vi "getItems.vi"(8 "error in (no error)":errorcluster, 11 "IFolder in":refnum<class "IFolder.lvclass">) -> (0 "error out":errorcluster, 2 "Components out":refnum<class "IComponent.lvclass">[](array[class]), 3 "IFolder out":refnum<class "IFolder.lvclass">)   [LabVIEW 2022 SP3, in "openDAQ.lvlib" / "IBaseObject.lvlib" / "IPropertyObject.lvlib" / "IComponent.lvlib" / "IFolder.lvlib" / "IFolder.lvclass"]
uses:
  <instrlib>/openDAQ/Public/Classes/IFolder/IFolder.lvclass
  C:/Program Files (x86)/National Instruments/LabVIEW 2022/instr.lib/openDAQ/Public/Classes/IBaseObject/IBaseObject.lvclass
  <instrlib>/openDAQ/Public/Classes/IComponent/IComponent.lvclass
  <instrlib>/openDAQ/Public/Classes/daqCoreTypes/IList/IList.lvclass
  <instrlib>/openDAQ/Public/Classes/IBaseObject/IBaseObject.lvclass/IBaseObject.ctl
  <instrlib>/openDAQ/Public/Classes/IBaseObject/Accessor/Read reference.vi
  <instrlib>/openDAQ/Public/Classes/IBaseObject/Accessor/Write reference.vi
  <instrlib>/openDAQ/Public/Classes/daqCoreTypes/IList/Polymorphic/getList/getComponentList.vi
  <instrlib>/openDAQ/Binaries/Windows/x86/copendaq32.dll
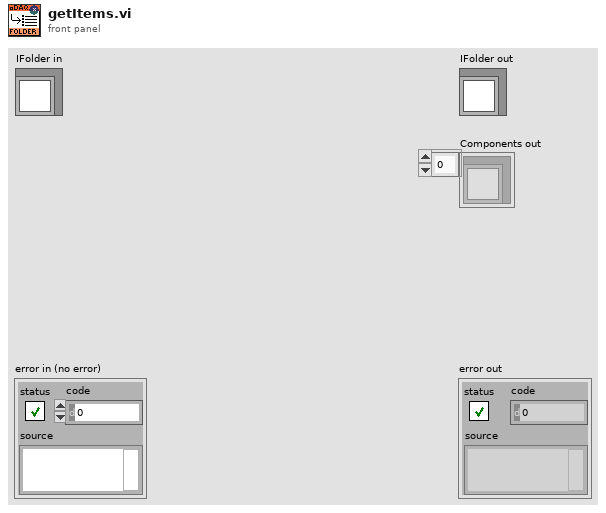
[diagram p1: front panel]
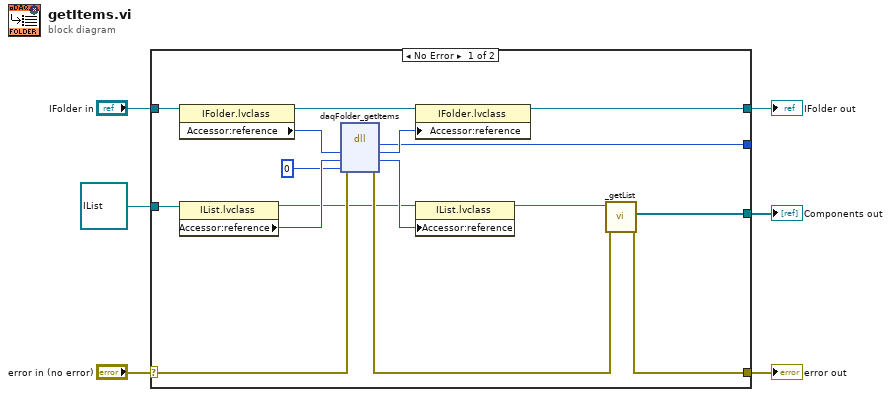
[diagram p0: block diagram]
diagram:
  n1 = case shown="No Error" "error in (no error)" {
    selector: "error in (no error)" -> [w21 w24]
    tunnel: [w13 w24] -> w5
    tunnel: [w10 w23] -> w3
    tunnel: "IFolder in" -> [w22 w23]
    tunnel: refnum<class "IList.lvclass"> refnum ("openDAQ.lvlib:daqCoreTypes.lvlib:IList.lvclass") -> [w20 _]
    tunnel: [w12 _] -> w1
    tunnel: [w8 _] -> _
    frame No Error {
      n2 = property class="IFolder.lvclass"(reference=w22) -> (reference out=w11:refnum<class "IFolder.lvclass">, "Accessor:reference"=w19:i64)  [unwired: 1 in, 1 out]
      n3 = property class="IList.lvclass"(reference=w20) -> (reference out=w9:refnum<class "IList.lvclass">, "Accessor:reference"=w18:i64)  [unwired: 1 in, 1 out]
      n4 = dll-call lib="C:/Program Files (x86)/National Instruments/LabVIEW 2022/instr.lib/openDAQ/Binaries/Windows/x86/copendaq*.*" fn="daqFolder_getItems"(error in=w21, "folder"=w19, "componentList"=w18, "searchFilter"=i64 0) -> (error out=w14:errorcluster, "return type"=w8:u32, "folder"=w17:i64, "componentList"=w16:i64)  [unwired: 3 in, 1 out]
      n5 = property class="IFolder.lvclass"(reference=w11, "Accessor:reference"=w17) -> (reference out=w10:refnum<class "IFolder.lvclass">)  [unwired: 1 in, 1 out]
      n6 = property class="IList.lvclass"(reference=w9, "Accessor:reference"=w16) -> (reference out=w15:refnum<class "IList.lvclass">)  [unwired: 1 in, 1 out]
      n7 = call-poly <instrlib>:"_getList.vi"("error in (no error)"=w14, "IList in"=w15) -> ("error out"=w13:errorcluster, "Components out"=w12:refnum<class "IComponent.lvclass">[])  [unwired: 8 in]
    }
    frame Error {
    }
  }
  "error out" <- w5
  "IFolder out" <- w3
  "Components out" <- w1
